vi "Temperature_DSP.vi"(1 "BIT 2":u16) -> (0 "Temperatura":ext)   [LabVIEW 2017]
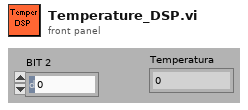
[diagram p1: front panel]
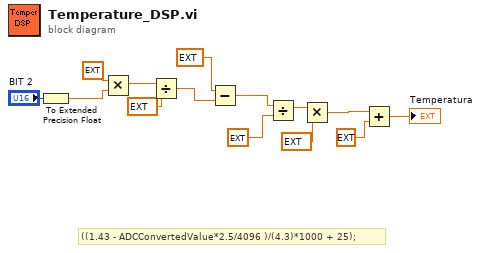
[diagram p0: block diagram]
diagram:
  # "((1.43 - ADCConvertedValue*2.5/4096 )/(4.3)*1000 + 25);"
  n1 = To Extended Precision Float(1:"BIT 2") -> (0:w7:ext)
  n2 = Multiply(x=ext 2.5, y=w7) -> (x*y=w4:ext)
  n3 = Divide(x=w4, y=ext 4095.0) -> (x/y=w9:ext)
  n4 = Subtract(x=ext 1.42999999999999999995, y=w9) -> (x-y=w10:ext)
  n5 = Divide(x=w10, y=ext 4.3000000000000000002) -> (x/y=w12:ext)
  n6 = Multiply(x=w12, y=ext 1000.0) -> (x*y=w2:ext)
  n7 = Add(x=w2, y=ext 25.0) -> (x+y=→"Temperatura":ext)
